vi "Read configuration.vi"(7 "force loading?":bool=TRUE, 8 "error in (no error)":errorcluster, 11 "Cascade512II in":refnum<class "DAQCascade512II.lvclass">) -> (0 "error out":errorcluster, 3 "Cascade512II out":refnum<class "DAQCascade512II.lvclass">)   [LabVIEW 2012, in "DAQCascade512II.lvclass"]
doc: "Reads the XML-based configuration file and populates the configuration cluster accordingly. Configuration file name is <component ID>.xml."
uses:
  DAQCascade512II.lvclass
  <vilib>/Distrio/Murmex/Murmex/Murmex.lvclass
  DAQCascade512II.lvclass/DAQCascade512II.ctl
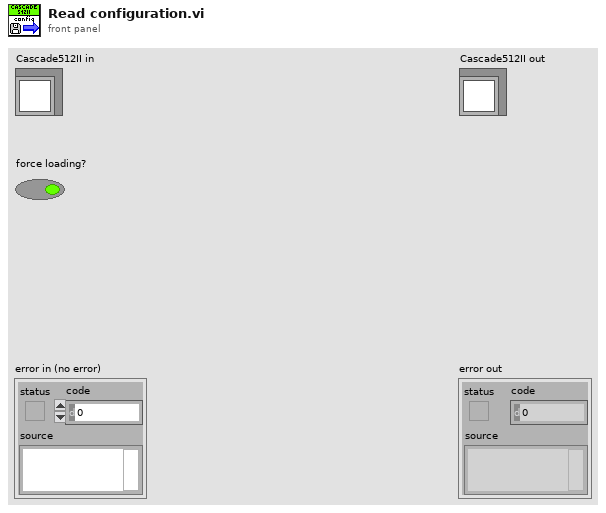
[diagram p1: front panel]
types:
  T1 = typedef "DAQCascade512II.lvclass/configuration cluster.ctl" = cluster{"Temperature":dbl, "Acquire / Focus Flag  of trigger":u32, "Number of Images fo Initializer":u32, "Data Type":u32, "Timing Mode of trigger ":u32}
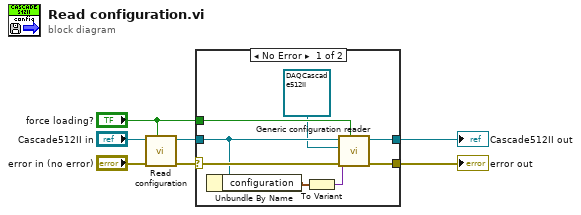
[diagram p0: block diagram]
diagram:
  n1 = call-parent "Read configuration.vi"("force loading?"="force loading?", "error in (no error)"="error in (no error)", "Murmex in"="Cascade512II in") -> ("error out"=w5:errorcluster, "Murmex out"=w3:refnum<class "DAQCascade512II.lvclass">)  [unwired: 7 in]
  n2 = case shown="No Error" w5 {
    selector: w5 -> [w15 w16]
    tunnel: "force loading?" -> [w13 _]
    tunnel: w3 -> [w11 w17]
    tunnel: [w14 w16] -> w2
    tunnel: [w12 w17] -> w1
    frame No Error {
      n3 = Unbundle By Name(w11) -> ("configuration"=w10:T1)
      n4 = To Variant(anything=w10) -> (Variant=w9:variant)
      n5 = call <vilib>:"Generic configuration reader.vi"("force loading?"=w13, "error in (no error)"=w15, "configuration cluster variant"=w9, "inheritance level"=refnum<class "DAQCascade512II.lvclass"> refnum ("DAQCascade512II"), "Murmex in"=w11) -> ("error out"=w14:errorcluster, "Murmex out"=w12:refnum<class "DAQCascade512II.lvclass">)  [unwired: 3 in, 2 out]
    }
    frame Error {
    }
  }
  "error out" <- w2
  "Cascade512II out" <- w1
